vi "Global_config.vi"() -> ()   [LabVIEW 2019]
panel:
  in  "val":cluster{"Scrip Path":path}
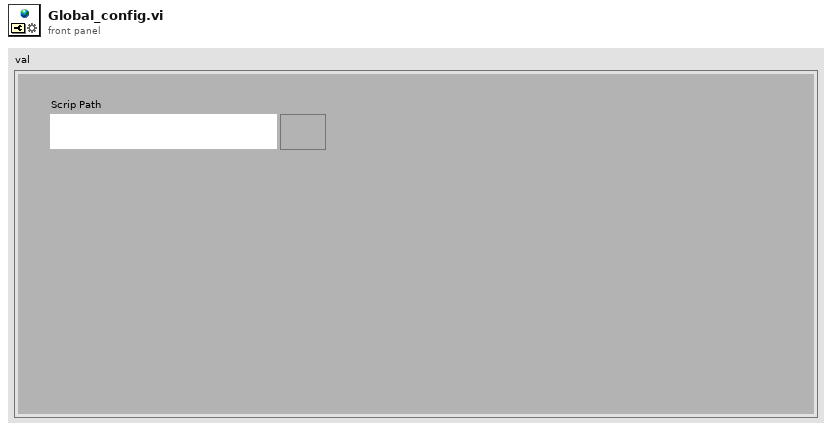
[diagram p1: front panel]
diagram:
